vi "Binary U8 to Digital Waveform.vi"(8 "error in (no error)":errorcluster, 9 "Time Division (0.0001 s)":dbl=0.0001, 10 "Compress Data (T: Enable)":bool=TRUE, 11 "Binary Array":i32[](array[numeric])) -> (0 "error out":errorcluster, 3 "Digital Waveform Graph":digitalwaveform(graph))   [LabVIEW 2013, in "Tektronix DPO MSO 2000 4000 Series.lvlib"]
doc: "Converts a binary array of unsigned integers to a digital waveform or set of digital data."
uses:
  Tektronix DPO MSO 2000 4000 Series.lvlib
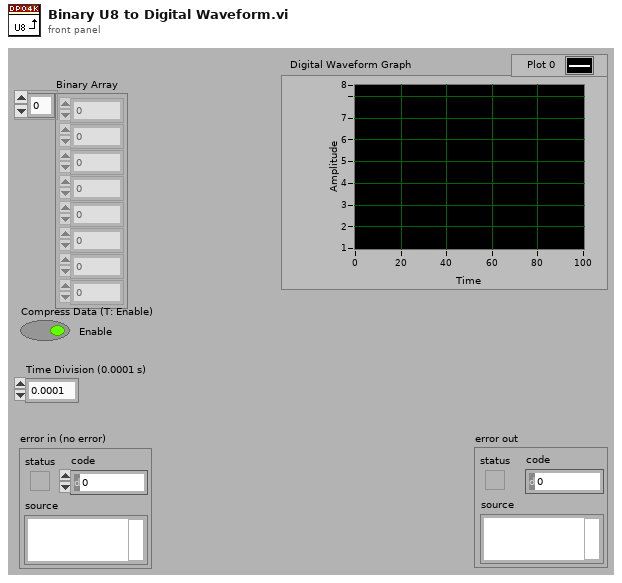
[diagram p1: front panel]
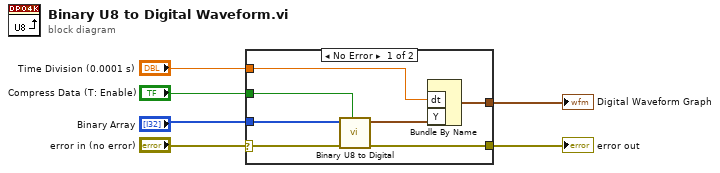
[diagram p0: block diagram]
diagram:
  n1 = case shown="No Error" "error in (no error)" {
    selector: "error in (no error)" -> [w10 w14]
    tunnel: "Binary Array" -> [w11 _]
    tunnel: [w9 w14] -> w5
    tunnel: [w13 _] -> w2
    tunnel: "Compress Data (T: Enable)" -> [w12 _]
    tunnel: "Time Division (0.0001 s)" -> [w7 _]
    frame No Error {
      n2 = call "Binary U8 to Digital.vi"("Compress Data (T: Enable)"=w12, "error in (no error)"=w10, "Binary Array"=w11) -> ("error out"=w9:errorcluster, "Digital Data"=w8:digitaldata)  [unwired: 7 in]
      n3 = Bundle By Name("dt"=w7, "Y"=w8) -> (w13:digitalwaveform)  [unwired: 1 in]
    }
    frame Error {
    }
  }
  "error out" <- w5
  "Digital Waveform Graph" <- w2
